vi "Move cursor to position.vi"(4 "error in":errorcluster, 5 "input main cluster":T1, 6 "Y":dbl, 7 "X":dbl) -> (0 "error out":errorcluster, 1 "output main cluster":T1)   [LabVIEW 2010]
uses:
  Main_cluster.ctl
  <vilib>/Utility/miscctls.llb/LVPointDoubleTypeDef.ctl
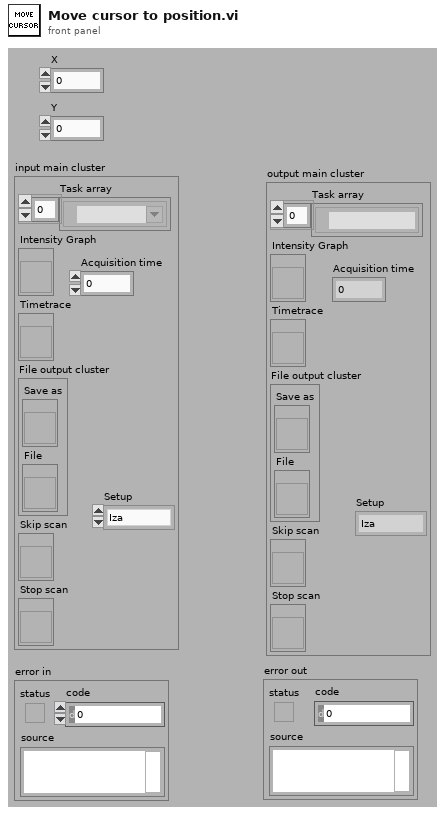
[diagram p1: front panel]
types:
  T1 = typedef "Main_cluster.ctl" = cluster{"Task array":refnum<k21>[], "Intensity Graph":refnum<vi>, "Timetrace":refnum<vi>, "File output cluster":cluster{"Save as":refnum<vi>, "File":refnum<vi>}, "Skip scan":refnum<vi>, "Stop scan":refnum<vi>, "Acquisition time":dbl, "Setup":enum16{"Iza", "Lukasz"}}
  T2 = typedef "LVPointDoubleTypeDef.ctl" = cluster{"X":dbl, "Y":dbl}
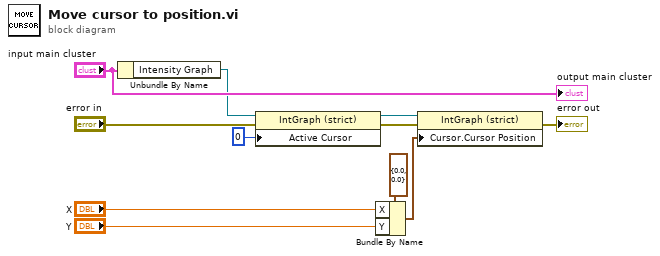
[diagram p0: block diagram]
diagram:
  n1 = Unbundle By Name("input main cluster") -> ("Intensity Graph"=w2:refnum<vi>)
  n2 = property on="Property Node" class="IntGraph (strict)"(reference=w2, error in="error in", "Active Cursor"=u32 0) -> (reference out=w1:refnum<vi>, error out=w11:errorcluster)
  n3 = Bundle By Name(cluster=T2 {"X"=0.0, "Y"=0.0} ("Cursor.Cursor Position"), "X"="X", "Y"="Y") -> (w9:T2)
  n4 = property on="Property Node" class="IntGraph (strict)"(reference=w1, error in=w11, "Cursor.Cursor Position"=w9) -> (error out=→"error out":errorcluster)  [unwired: 1 out]
  "output main cluster" <- "input main cluster"
